vi "Load State Machine.vi"   [LabVIEW 2013]
uses:
  typedefs/singleUseSubstate.ctl
  <vilib>/Rock Robotics/WPI/Solenoid/WPI_SolenoidValue.ctl
  typedefs/fg_typedef.ctl
  typedefs/DevRef Type.ctl
  typedefs/subStates.ctl
  <vilib>/Rock Robotics/WPI/Solenoid/WPI_SolenoidGetEnum.vi
panel:
  # "A State Machine to Handle Loading for Either High or Low Goal Shots"
types:
  T1 = typedef "DevRef Type.ctl" = enum16{"Shooter Solenoid", "Latch Solenoid", "Right Up Sensor", "Right Down Sensor", "Hold Sensor", "2 Ball Switch", "Arm Encoder"}
  T2 = typedef "fg_typedef.ctl" = enum16{"Get", "Set"}
  T3 = typedef "WPI_SolenoidValue.ctl" = enum16{"Off", "On", "Forward", "Reverse"}
  T4 = typedef "singleUseSubstate.ctl" = enum16{"null", "wait", "shift high", "shift low", "extend shooter", "retract shooter", "latch", "unlatch", "end"}
  T5 = typedef "subStates.ctl" = enum16{"null", "wait", "driver control", "auto", "manual override", "hold position", "rotate", "pickup", "pass", "load", "goto shoot", "shoot high goal", "shoot low goal", "cancel arm", "cancel shooter", "end", "test"}
  T6 = typedef "WPI_SolenoidDevRef.ctl" = cluster{"DevStatus":errorcluster, "Solenoid Module":T7, "Forward Solenoid Channel":T8, "Reverse Solenoid Channel":T8}
  T7 = typedef "FPGA_TypedefSolenoidModule.ctl" = enum16{"Solenoid Module 1", "Solenoid Module 2"}
  T8 = typedef "WPI_SolenoidChannel.ctl" = enum8{"Solenoid 1", "Solenoid 2", "Solenoid 3", "Solenoid 4", "Solenoid 5", "Solenoid 6", "Solenoid 7", "Solenoid 8", "Invalid"}
  T9 = typedef "WPI_DigitalInputDevRef.ctl" = cluster{"DevStatus":errorcluster, "DIO Channel":T10, "Digital Module":T11}
  T10 = typedef "FPGA_DIOChannel.ctl" = enum8{"DIO 1", "DIO 2", "DIO 3", "DIO 4", "DIO 5", "DIO 6", "DIO 7", "DIO 8", "DIO 9", "DIO 10", "DIO 11", "DIO 12", "DIO 13", "DIO 14", "Invalid"}
  T11 = typedef "FPGA_TypedefDigitalModule.ctl" = enum16{"Digital Module 1", "Digital Module 2"}
  T12 = typedef "WPI_EncoderDevRef.ctl" = cluster{"DevStatus":errorcluster, "EncoderIndex":T13, "CounterIndex":T14, "DistancePerCount":dbl, "Decoding Type":T15}
  T13 = typedef "FPGA_EncoderIdx.ctl" = enum8{"Enc 0", "Enc 1", "Enc 2", "Enc 3", "Invalid"}
  T14 = typedef "FPGA_CounterCtrSystemIndex.ctl" = enum8{"Ctr 0", "Ctr 1", "Ctr 2", "Ctr 3", "Ctr 4", "Ctr 5", "Ctr 6", "Ctr 7", "Invalid"}
  T15 = typedef "WPI_EncoderType.ctl" = enum16{"1x", "2x", "4x"}
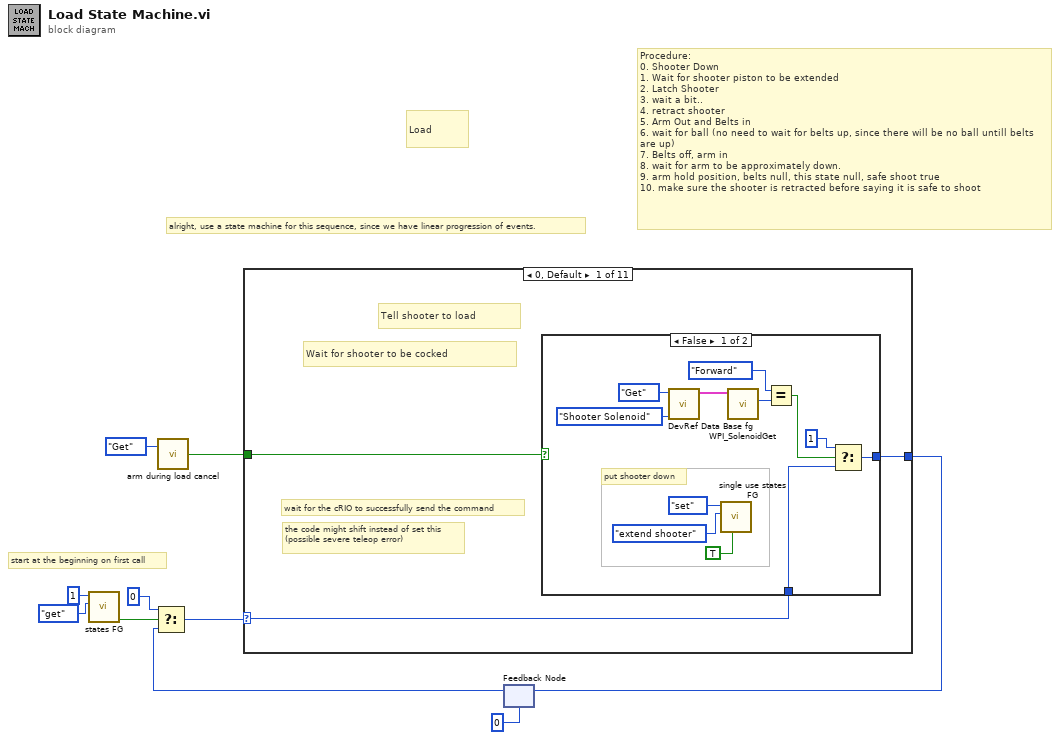
[diagram p0: block diagram]
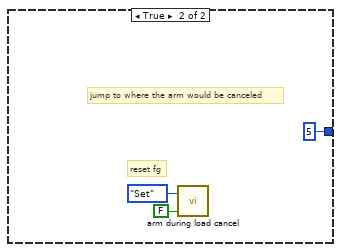
[diagram p2: hidden frame]
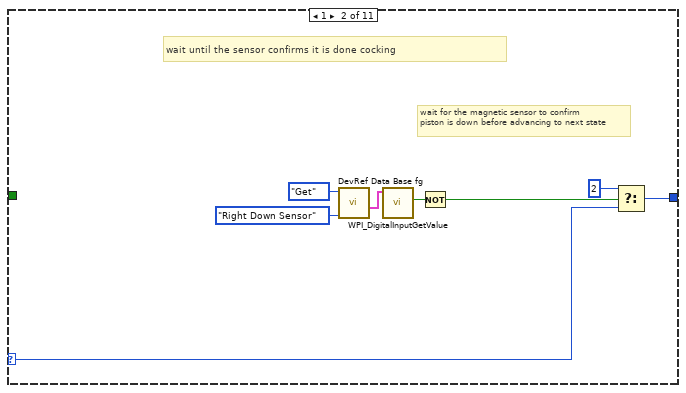
[diagram p3: hidden frame]
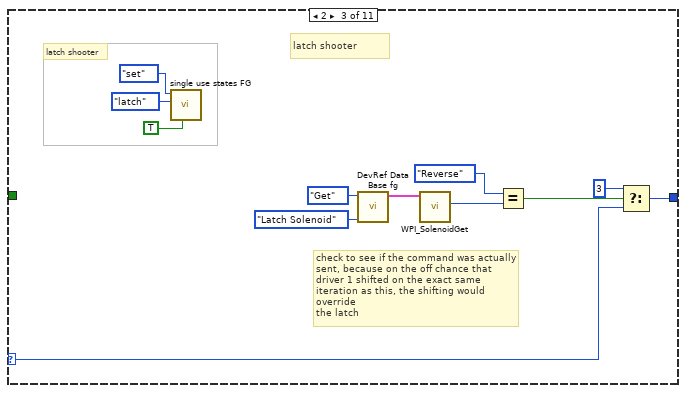
[diagram p4: hidden frame]
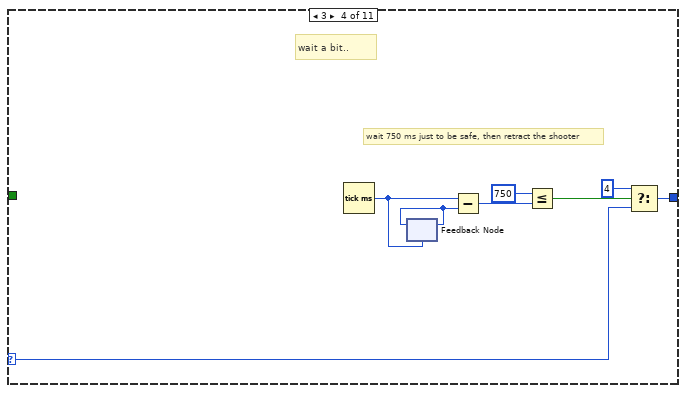
[diagram p5: hidden frame]
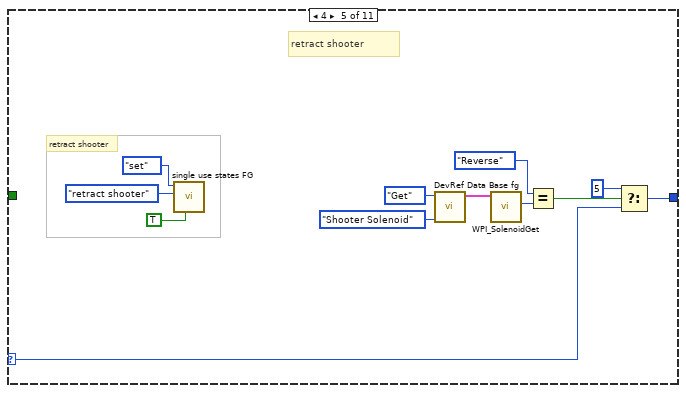
[diagram p6: hidden frame]
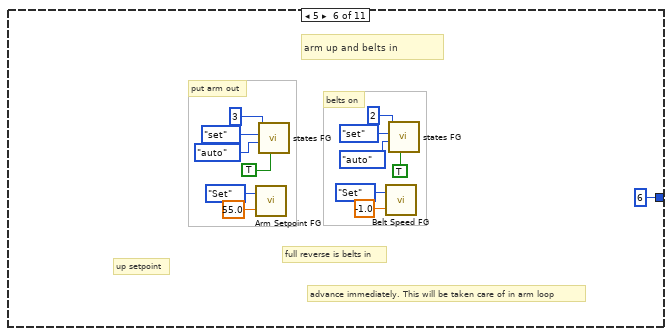
[diagram p7: hidden frame]
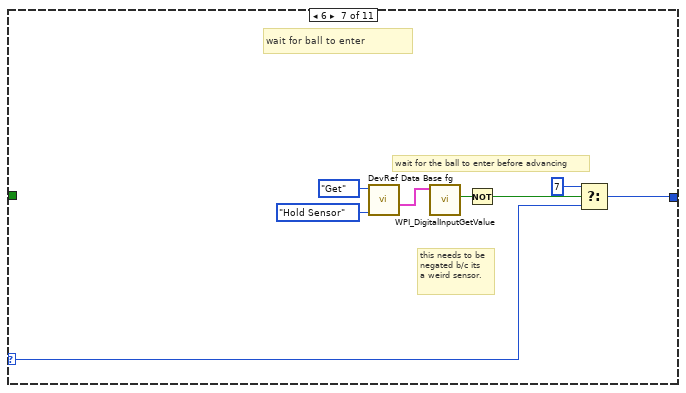
[diagram p8: hidden frame]
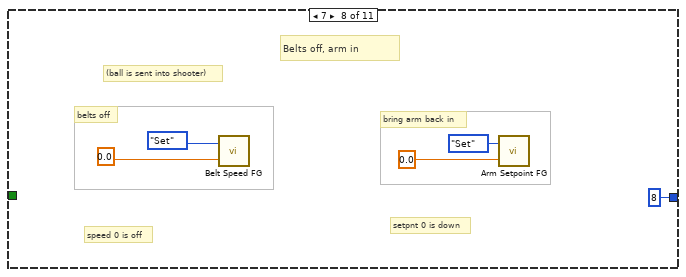
[diagram p9: hidden frame]
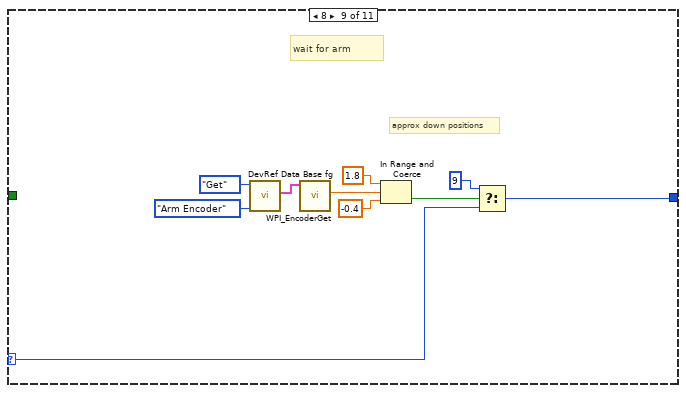
[diagram p10: hidden frame]
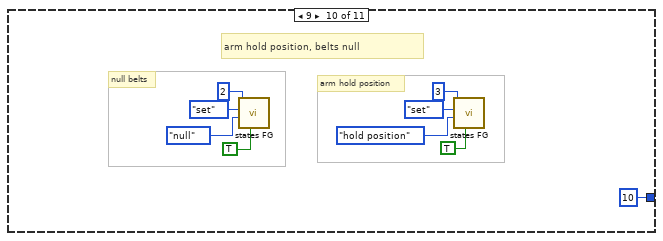
[diagram p11: hidden frame]
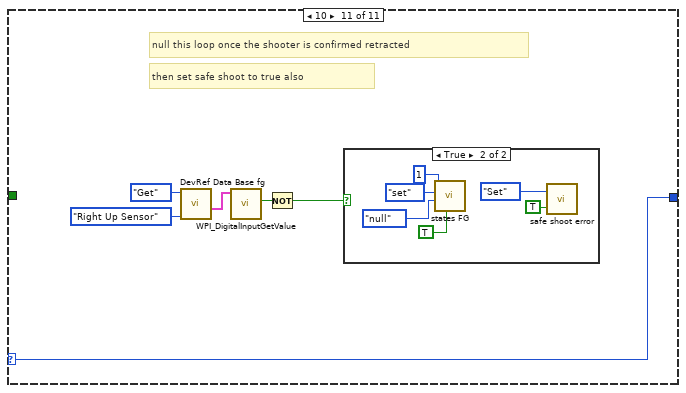
[diagram p12: hidden frame]
diagram:
  # "start at the beginning on first call"
  # "Load"
  # "Procedure: \n0. Shooter Down \n1. Wait for shooter piston to be extended\n2. Latch Shooter\n3. wait a bit..\n4. retract shooter\n5. Arm Out and Belts in\n6. wait for ball (no need to wait for belts up, since there will be no ball untill belts are up)\n7. Belts off, arm in\n8. wait for arm to be approximately down.\n9. arm hold position, belts null, this state null, safe shoot true\n10. make sure the shooter is retracted before saying it is safe to shoot"
  # "alright, use a state machine for this sequence, since we have linear progression of events."
  n1 = call "states FG.vi"("menu (get)"=enum16{"set", "get"}."get", "Loop ID"=1) -> ("first call?"=w3:bool)  [unwired: 6 in, 3 out]
  n2 = call "arm during load cancel.vi"("Mode"=enum16{"Get", "Set", "Teleop Set"}."Get") -> ("Arm Canceled During Load"=w1:bool)  [unwired: 1 in]
  n3 = feedback #1(u8 0) -> (w4:u8)
  n4 = Select(t=u8 0, s=w3, f=w4) -> (s? t:f=w6:u8)
  n5 = case shown="0, Default" w6 {
    selector: w6 -> [w12 w34 w44 w50 w65 _ w87 _ w100 _ w119]
    tunnel: [w13 w33 w45 w52 w64 u8 6 ("t") w86 u8 8 ("t") w99 u8 10 ("t") w119] -> w9
    tunnel: w1 -> [w11 _ _ _ _ _ _ _ _ _ _]
    frame 0, Default {
      # "the code might shift instead of set this\n(possible severe teleop error)"
      # "Wait for shooter to be cocked"
      # "wait for the cRIO to successfully send the command"
      # "Tell shooter to load"
      n6 = case shown="False" w11 {
        tunnel: [w22 u8 5 ("t")] -> w13
        tunnel: w12 -> [w21 _]
        frame False {
          # "put shooter down"
          n7 = call "DevRef Data Base fg.vi"("DevRef to Get"=DevRef_Type."Shooter Solenoid", "Menu"=fg_typedef."Get") -> ("Selected Solenoid"=w20:T6)  [unwired: 2 in, 5 out]
          n8 = call "single use states FG.vi"("exit in"=TRUE, "substate"=singleUseSubstate."extend shooter", "menu (get)"=enum16{"set", "get"}."set") -> ()  [unwired: 5 in, 4 out]
          n9 = call-poly <vilib>:"WPI_SolenoidGet.vi"("SolenoidDevRef"=w20) -> ("Value"=w19:T3)  [unwired: 8 in, 2 out]
          n10 = Equal?(x=WPI_SolenoidValue."Forward", y=w19) -> (x = y?=w17:bool)
          n11 = Select(t=u8 1, s=w17, f=w21) -> (s? t:f=w22:u8)
        }
        frame True {
          # "reset fg"
          # "jump to where the arm would be canceled"
          n12 = call "arm during load cancel.vi"("Arm Canceled During Load?"=FALSE, "Mode"=enum16{"Get", "Set", "Teleop Set"}."Set") -> ()  [unwired: 1 out]
        }
      }
    }
    frame 1 {
      # "wait for the magnetic sensor to confirm \npiston is down before advancing to next state"
      # "wait until the sensor confirms it is done cocking"
      n13 = call "DevRef Data Base fg.vi"("DevRef to Get"=DevRef_Type."Right Down Sensor", "Menu"=fg_typedef."Get") -> ("Selected Sensor"=w35:T9)  [unwired: 2 in, 5 out]
      n14 = call <vilib>:"WPI_DigitalInputGetValue.vi"("DigitalInputDevRef"=w35) -> ("Value"=w36:bool)  [unwired: 8 in, 2 out]
      n15 = Not(x=w36) -> (.not. x?=w31:bool)
      n16 = Select(t=u8 2, s=w31, f=w34) -> (s? t:f=w33:u8)
    }
    frame 2 {
      # "latch shooter"
      # "check to see if the command was actually\nsent, because on the off chance that\ndriver 1 shifted on the exact same\niteration as this, the shifting would override\nthe latch"
      # "latch shooter"
      n17 = call "single use states FG.vi"("exit in"=TRUE, "substate"=singleUseSubstate."latch", "menu (get)"=enum16{"set", "get"}."set") -> ()  [unwired: 5 in, 4 out]
      n18 = call "DevRef Data Base fg.vi"("DevRef to Get"=DevRef_Type."Latch Solenoid", "Menu"=fg_typedef."Get") -> ("Selected Solenoid"=w43:T6)  [unwired: 2 in, 5 out]
      n19 = call-poly <vilib>:"WPI_SolenoidGet.vi"("SolenoidDevRef"=w43) -> ("Value"=w42:T3)  [unwired: 8 in, 2 out]
      n20 = Equal?(x=WPI_SolenoidValue."Reverse" ("Value"), y=w42) -> (x = y?=w40:bool)
      n21 = Select(t=u8 3, s=w40, f=w44) -> (s? t:f=w45:u8)
    }
    frame 3 {
      # "wait a bit.."
      # "wait 750 ms just to be safe, then retract the shooter"
      n22 = Tick Count (ms)() -> (millisecond timer value=w54:u32)
      n23 = feedback #2(w54) -> (w55:u32)
      n24 = feedback-in #2(w55) -> ()
      n25 = Subtract(x=w54, y=w55) -> (x-y=w53:u32)
      n26 = Less Or Equal?(x=u32 750, y=w53) -> (x <= y?=w51:bool)
      n27 = Select(t=u8 4, s=w51, f=w50) -> (s? t:f=w52:u8)
    }
    frame 4 {
      # "retract shooter"
      # "retract shooter"
      n28 = call "single use states FG.vi"("exit in"=TRUE, "substate"=singleUseSubstate."retract shooter", "menu (get)"=enum16{"set", "get"}."set") -> ()  [unwired: 5 in, 4 out]
      n29 = call "DevRef Data Base fg.vi"("DevRef to Get"=DevRef_Type."Shooter Solenoid", "Menu"=fg_typedef."Get") -> ("Selected Solenoid"=w63:T6)  [unwired: 2 in, 5 out]
      n30 = call-poly <vilib>:"WPI_SolenoidGet.vi"("SolenoidDevRef"=w63) -> ("Value"=w62:T3)  [unwired: 8 in, 2 out]
      n31 = Equal?(x=WPI_SolenoidValue."Reverse", y=w62) -> (x = y?=w60:bool)
      n32 = Select(t=u8 5, s=w60, f=w65) -> (s? t:f=w64:u8)
    }
    frame 5 {
      # "full reverse is belts in"
      # "belts on"
      # "up setpoint"
      # "arm up and belts in"
      # "advance immediately. This will be taken care of in arm loop"
      # "put arm out"
      n33 = call "Arm Setpoint FG.vi"("Setpoint In"=55.0, "Menu"=fg_typedef."Set") -> ()  [unwired: 1 out]
      n34 = call "states FG.vi"("exit in"=TRUE, "subState in"=subStates."auto", "menu (get)"=enum16{"set", "get"}."set", "Loop ID"=3) -> ()  [unwired: 4 in, 4 out]
      n35 = call "Belt Speed FG.vi"("Speed In"=-1.0 ("Setpoint In"), "Menu"=fg_typedef."Set") -> ()  [unwired: 1 out]
      n36 = call "states FG.vi"("exit in"=TRUE, "subState in"=subStates."auto", "menu (get)"=enum16{"set", "get"}."set", "Loop ID"=2) -> ()  [unwired: 4 in, 4 out]
    }
    frame 6 {
      # "this needs to be\nnegated b/c its\na weird sensor."
      # "wait for the ball to enter before advancing"
      # "wait for ball to enter"
      n37 = call "DevRef Data Base fg.vi"("DevRef to Get"=DevRef_Type."Hold Sensor", "Menu"=fg_typedef."Get") -> ("Selected Sensor"=w85:T9)  [unwired: 2 in, 5 out]
      n38 = call <vilib>:"WPI_DigitalInputGetValue.vi"("DigitalInputDevRef"=w85) -> ("Value"=w89:bool)  [unwired: 8 in, 2 out]
      n39 = Not(x=w89) -> (.not. x?=w88:bool)
      n40 = Select(t=u8 7, s=w88, f=w87) -> (s? t:f=w86:u8)
    }
    frame 7 {
      # "bring arm back in"
      # "setpnt 0 is down"
      # "speed 0 is off"
      # "Belts off, arm in"
      # "(ball is sent into shooter)"
      # "belts off"
      n41 = call "Belt Speed FG.vi"("Speed In"=0.0 ("Setpoint In"), "Menu"=fg_typedef."Set") -> ()  [unwired: 1 out]
      n42 = call "Arm Setpoint FG.vi"("Setpoint In"=0.0, "Menu"=fg_typedef."Set") -> ()  [unwired: 1 out]
    }
    frame 8 {
      # "approx down positions"
      # "wait for arm"
      n43 = call "DevRef Data Base fg.vi"("DevRef to Get"=DevRef_Type."Arm Encoder", "Menu"=fg_typedef."Get") -> ("Selected Encoder"=w104:T12)  [unwired: 2 in, 5 out]
      n44 = call <vilib>:"WPI_EncoderGet.vi"("EncoderDevRef"=w104) -> ("Distance"=w103:dbl)  [unwired: 5 in, 5 out]
      n45 = In Range and Coerce(upper limit=1.8, x=w103, lower limit=-0.4) -> (In Range?=w97:bool)  [unwired: 1 out]
      n46 = Select(t=u8 9, s=w97, f=w100) -> (s? t:f=w99:u8)
    }
    frame 9 {
      # "arm hold position, belts null"
      # "arm hold position"
      # "null belts"
      n47 = call "states FG.vi"("exit in"=TRUE, "subState in"=subStates."null", "menu (get)"=enum16{"set", "get"}."set", "Loop ID"=2) -> ()  [unwired: 4 in, 4 out]
      n48 = call "states FG.vi"("exit in"=TRUE, "subState in"=subStates."hold position", "menu (get)"=enum16{"set", "get"}."set", "Loop ID"=3) -> ()  [unwired: 4 in, 4 out]
    }
    frame 10 {
      # "then set safe shoot to true also"
      # "null this loop once the shooter is confirmed retracted"
      n49 = call "DevRef Data Base fg.vi"("DevRef to Get"=DevRef_Type."Right Up Sensor", "Menu"=fg_typedef."Get") -> ("Selected Sensor"=w118:T9)  [unwired: 2 in, 5 out]
      n50 = call <vilib>:"WPI_DigitalInputGetValue.vi"("DigitalInputDevRef"=w118) -> ("Value"=w117:bool)  [unwired: 8 in, 2 out]
      n51 = Not(x=w117) -> (.not. x?=w116:bool)
      n52 = case shown="True" w116 {
        frame False {
        }
        frame True {
          n53 = call "states FG.vi"("exit in"=TRUE, "subState in"=subStates."null", "menu (get)"=enum16{"set", "get"}."set", "Loop ID"=1) -> ()  [unwired: 4 in, 4 out]
          n54 = call "safe shoot error.vi"("Can Shoot Safely?"=TRUE, "Menu"=fg_typedef."Set") -> ()  [unwired: 1 out]
        }
      }
    }
  }
  n55 = feedback-in #1(w9) -> ()
